vi "Chamber_control_Apr_ 2018.vi"() -> ()   [LabVIEW 2014]
doc: "This template is for the Queued Message Handler design pattern.\n\nThe Event Handling Loop generates messages based on user interface actions.\n\nThe Message Handling Loop processes messages generated by the Event Handling Loop, or by other messages. The messages are string values, so new messages can be added easily to the Message Cases case structure in the Message Handling Loop. Each message cluster can also provide an optional value for Message Data, which is a variant that can be converted to whatever message-specific data is required."
uses:
  <vilib>/Analysis/baseanly.llb/Mean (DBL).vi
  <vilib>/Instr/_visa.llb/VISA Configure Serial Port (Instr).vi
  Environmental Chamber LabVIEW and Instruments/Drivers and Software/Keithley 2100 Series/Public/Configure/Configure 2 Wire Resistance.vi
  <vilib>/Utility/file.llb/Read From Spreadsheet File (string).vi
  <vilib>/Utility/file.llb/Write To Spreadsheet File (string).vi
  Environmental Chamber LabVIEW and Instruments/Drivers and Software/LabVIEW 8.2 Drivers/keithley_24xx/Keithley 24XX/Public/Data/Read (Single Point).vi
  Environmental Chamber LabVIEW and Instruments/Drivers and Software/keithley_6430/Keithley 6430/Public/Data/Read (Single Point).vi
  Environmental Chamber LabVIEW and Instruments/Drivers and Software/keithley_6430/Keithley 6430/Keithley 6430.lvlib
  Environmental Chamber LabVIEW and Instruments/Drivers and Software/Keithley 2100 Series/Keithley 2100 Series.lvlib
  Environmental Chamber LabVIEW and Instruments/Drivers and Software/keithley_24xx/Keithley 24XX/Keithley 24XX.lvlib
  <vilib>/Analysis/NI_AALBase.lvlib
panel:
  out "Resistance":sgl format="%#_6e"
  in  "K2420 DC bias (V)":dbl=0.05
  in  "SYSTEM CONTROL":T1={"valve % open"=0.0, "Desired pressure"=0.0, "set Vapor sccm"=0.0, "set Gas sccm"=0.0, "Valve mode"=enum."% Open", "Pressure Mode"=enum."Abs. pressure", "analyte partial pressure"=23.8, "Actual"=0.0, "Read pressure (Torr)"=0.0, "Read vapor flow (sccm)"=0.0, "Read gas flow (sccm)"=0.0, "Save now"=FALSE, "Stop after seq."=TRUE, "Turbo pump\nauto on"=TRUE, "Integrate points"=0} caption="Pressure settings" {"Integrate points" min=0 max=100 step=1; "analyte partial pressure" min=0.0 max=100.0 step=5.0; "set Gas sccm" min=0 max=200 step=5; "set Vapor sccm" min=0 max=200 step=5; "Desired pressure" min=0.0 max=760.0 step=5.0; "valve % open" min=0.0 max=100.0 step=5.0 format="%#_2f"}
  in  "SAVE SAMPLE / ANALYTE NAMES":T2={"QCM1"="", "QCM2"="", "QCM3"="", "QCM4"="broken", "QCM5"="NOT WORKING", "QCM6"="", "SRS"="bareAu", "K-2420"="", "K-6430"="", "K-2100"="", "Gas"="NOT WORKING", "Vapor"="H2O", "Notes"=""} caption="Save samplffe names"
  in  "Clear all charts":bool
  out "K-6430":dbl(graph)
  out "K-2420":dbl(graph)
  out "File":path caption="DATA FILE"
  in  "Stop":bool
  out "QCM plot":T3(graph)
  out "K-2100":dbl(graph)
  out "State date/time":string caption="Program start time"
  out "J-KEM temp":dbl(graph)
  out "saving data?":bool
  out "pressure chart":dbl(graph)
  out "arduino qcm stack plot":T4(graph)
  in  "SEQUENCE":T5 {"preview" items=["pressure", "gas flow", "vapor flow", "bias"]}
  # "100"
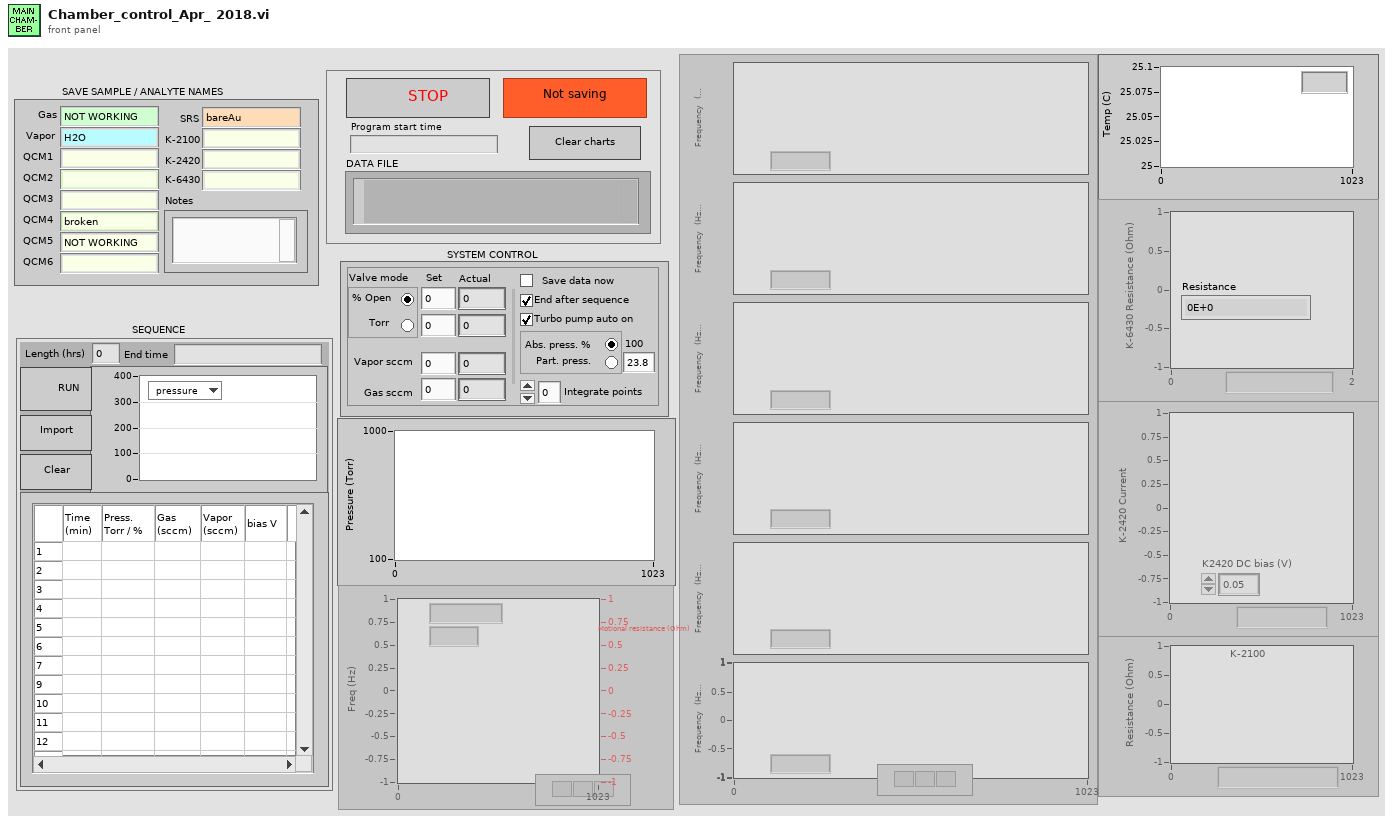
[diagram p1: front panel]
types:
  T1 = cluster{"valve % open":dbl, "Desired pressure":dbl, "set Vapor sccm":sgl, "set Gas sccm":sgl, "Valve mode":enum32{"% Open", "Torr "}, "Pressure Mode":enum32{"Abs. pressure", " Part. pressure"}, "analyte partial pressure":dbl, "Actual":dbl, "Read pressure (Torr)":dbl, "Read vapor flow (sccm)":dbl, "Read gas flow (sccm)":dbl, "Save now":bool, "Stop after seq.":bool, "Turbo pump\nauto on":bool, "Integrate points":i32}
  T2 = cluster{"QCM1":string, "QCM2":string, "QCM3":string, "QCM4":string, "QCM5":string, "QCM6":string, "SRS":string, "K-2420":string, "K-6430":string, "K-2100":string, "Gas":string, "Vapor":string, "Notes":string}
  T3 = cluster{"Frequency out":dbl, "Resistance out":dbl}
  T4 = cluster{"[0]":dbl, "[1]":dbl, "[2]":dbl, "[3]":dbl, "[4]":dbl, "[5]":dbl}
  T5 = cluster{"Run Sequence":bool, "User-defined\nsequence":string[][], "preview":u16, "Sequence\npreview":cluster{dbl[], dbl[]}[], "Clear sequence":bool, "Import sequence file":bool, "Length (hrs)":dbl, "End time":string}
  T6 = cluster{"Keithley 6430":bool, "J-KEM":bool, "Keithley 2420":bool, "Keithley 2100":bool, "SRS QCM":bool, "Pressure control":bool, "Arduino":bool}
  T7 = enum16{"open", "replace", "create", "open or create", "replace or create", "replace or create with confirmation"}
  T8 = cluster{"Arduino 1":refnum<visa-resource-name>, "Arduino 2":refnum<visa-resource-name>, "Arduino 3":refnum<visa-resource-name>, "Arduino 4":refnum<visa-resource-name>, "Arduino 5":refnum<visa-resource-name>, "Arduino 6":refnum<visa-resource-name>}
  T9 = enum8{"Enabled", "Disabled", "Disabled and Grayed Out"}
  T10 = cluster{"[0]":string, "[1]":string, "[2]":string, "[3]":string, "[4]":string, "[5]":string}
  T11 = cluster{"[0]":dbl, "[1]":dbl, "[2]":dbl, "[3]":dbl, "[4]":dbl, "[5]":dbl}[]
  T12 = cluster{"Frequency out":dbl, "Resistance out":dbl}[]
  T13 = cluster{"VISA resource name":refnum<visa-resource-name>, "error out":errorcluster, bool}
  T14 = cluster{"VISA resource name out":refnum<visa-resource-name>, "error out":errorcluster, bool}
  T15 = cluster{bool, "task out":refnum<k21>, "error out":errorcluster, "task out":refnum<k21>, "error out":errorcluster, "turbo pump":refnum<visa-resource-name>, "error out":errorcluster}
  T16 = cluster{bool, "task out":refnum<k21>, "error out":errorcluster, "task out":refnum<k21>, "error out":errorcluster, "VISA resource name out":refnum<visa-resource-name>, "error out":errorcluster}
  T17 = cluster{bool, "VISA resource name":refnum<visa-resource-name>, "error out":errorcluster}
  T18 = cluster{bool, "VISA resource name out":refnum<visa-resource-name>, "error out":errorcluster}
  T19 = cluster{bool, "VISA in":refnum<visa-resource-name>, "error out":errorcluster}
  T20 = cluster{bool, "VISA out":refnum<visa-resource-name>, "error out":errorcluster}
  T21 = cluster{"Arduino address":refnum<visa-resource-name>, "error in (no error)":errorcluster, "Arduino address 2":refnum<visa-resource-name>, "error in (no error) 2":errorcluster, "Arduino address 3":refnum<visa-resource-name>, "error in (no error) 3":errorcluster, "Arduino address 4":refnum<visa-resource-name>, "error in (no error) 4":errorcluster, "Arduino address 5":refnum<visa-resource-name>, "error in (no error) 5":errorcluster, "Arduino address 6":refnum<visa-resource-name>, "error in (no error) 6":errorcluster, "arduinos on?":bool}
  T22 = cluster{string[][], path, "data headers":string[]}
  T23 = cluster{"valve % open":dbl, "Desired pressure":dbl, "set Vapor sccm":sgl, "set Gas sccm":sgl, "Valve mode":enum32{"% Open", "Torr "}, "Pressure Mode":enum32{"Abs. pressure", " Part. pressure"}, "analyte partial pressure":dbl}
  T24 = cluster{"User-defined\nsequence":string[][], "Present (s)":dbl, "current  step # in":i32, "sequence end time in":timestamp}
  T25 = cluster{"current  step # in":i32, "sequence end time in":timestamp, "Boolean":bool}
  T26 = cluster{"press/RH/gas/vapor":cluster{"pressure":string, "RH":string, "gas flow":string, "vapor flow":string}, "Cluster":cluster{"Valve position (%)":dbl, "read pressure":dbl, "read vapor flow":dbl, "read gas flow":dbl}}
  T27 = cluster{"Boolean":bool, "task out":refnum<k21>, "error out":errorcluster, "task out":refnum<k21>, "error out":errorcluster, "VISA resource name out":refnum<visa-resource-name>, "error out":errorcluster}
  T28 = cluster{"t":string, "delta t":string, "p":string, "delta p":string}
  T29 = cluster{"pressure":string, "RH":string, "gas flow":string, "vapor flow":string}
  T30 = cluster{"Valve position (%)":dbl, "read pressure":dbl, "read vapor flow":dbl, "read gas flow":dbl}
  T31 = cluster{"Boolean":bool, "VISA resource name out":refnum<visa-resource-name>, "error out":errorcluster}
  T32 = cluster{"Boolean":bool, "VISA out":refnum<visa-resource-name>, "error out":errorcluster}
  T33 = cluster{"Boolean":bool, "Arduino address":refnum<visa-resource-name>, "error in (no error)":errorcluster, "Arduino address 2":refnum<visa-resource-name>, "error in (no error) 2":errorcluster, "Arduino address 3":refnum<visa-resource-name>, "error in (no error) 3":errorcluster, "Arduino address 4":refnum<visa-resource-name>, "error in (no error) 4":errorcluster, "Arduino address 5":refnum<visa-resource-name>, "error in (no error) 5":errorcluster, "Arduino address 6":refnum<visa-resource-name>, "error in (no error) 6":errorcluster}
  T34 = cluster{"arduino addresses out":cluster{"Boolean":bool, "Arduino address":refnum<visa-resource-name>, "error in (no error)":errorcluster, "Arduino address 2":refnum<visa-resource-name>, "error in (no error) 2":errorcluster, "Arduino address 3":refnum<visa-resource-name>, "error in (no error) 3":errorcluster, "Arduino address 4":refnum<visa-resource-name>, "error in (no error) 4":errorcluster, "Arduino address 5":refnum<visa-resource-name>, "error in (no error) 5":errorcluster, "Arduino address 6":refnum<visa-resource-name>, "error in (no error) 6":errorcluster}, cluster{bool, "VISA resource name out":refnum<visa-resource-name>, "error out":errorcluster}, "Address out":cluster{"Boolean":bool, "VISA resource name out":refnum<visa-resource-name>, "error out":errorcluster}, cluster{bool, "VISA resource name out":refnum<visa-resource-name>, "error out":errorcluster}, cluster{bool, "VISA resource name out":refnum<visa-resource-name>, "error out":errorcluster}, "SRS address out":cluster{"Boolean":bool, "VISA out":refnum<visa-resource-name>, "error out":errorcluster}}
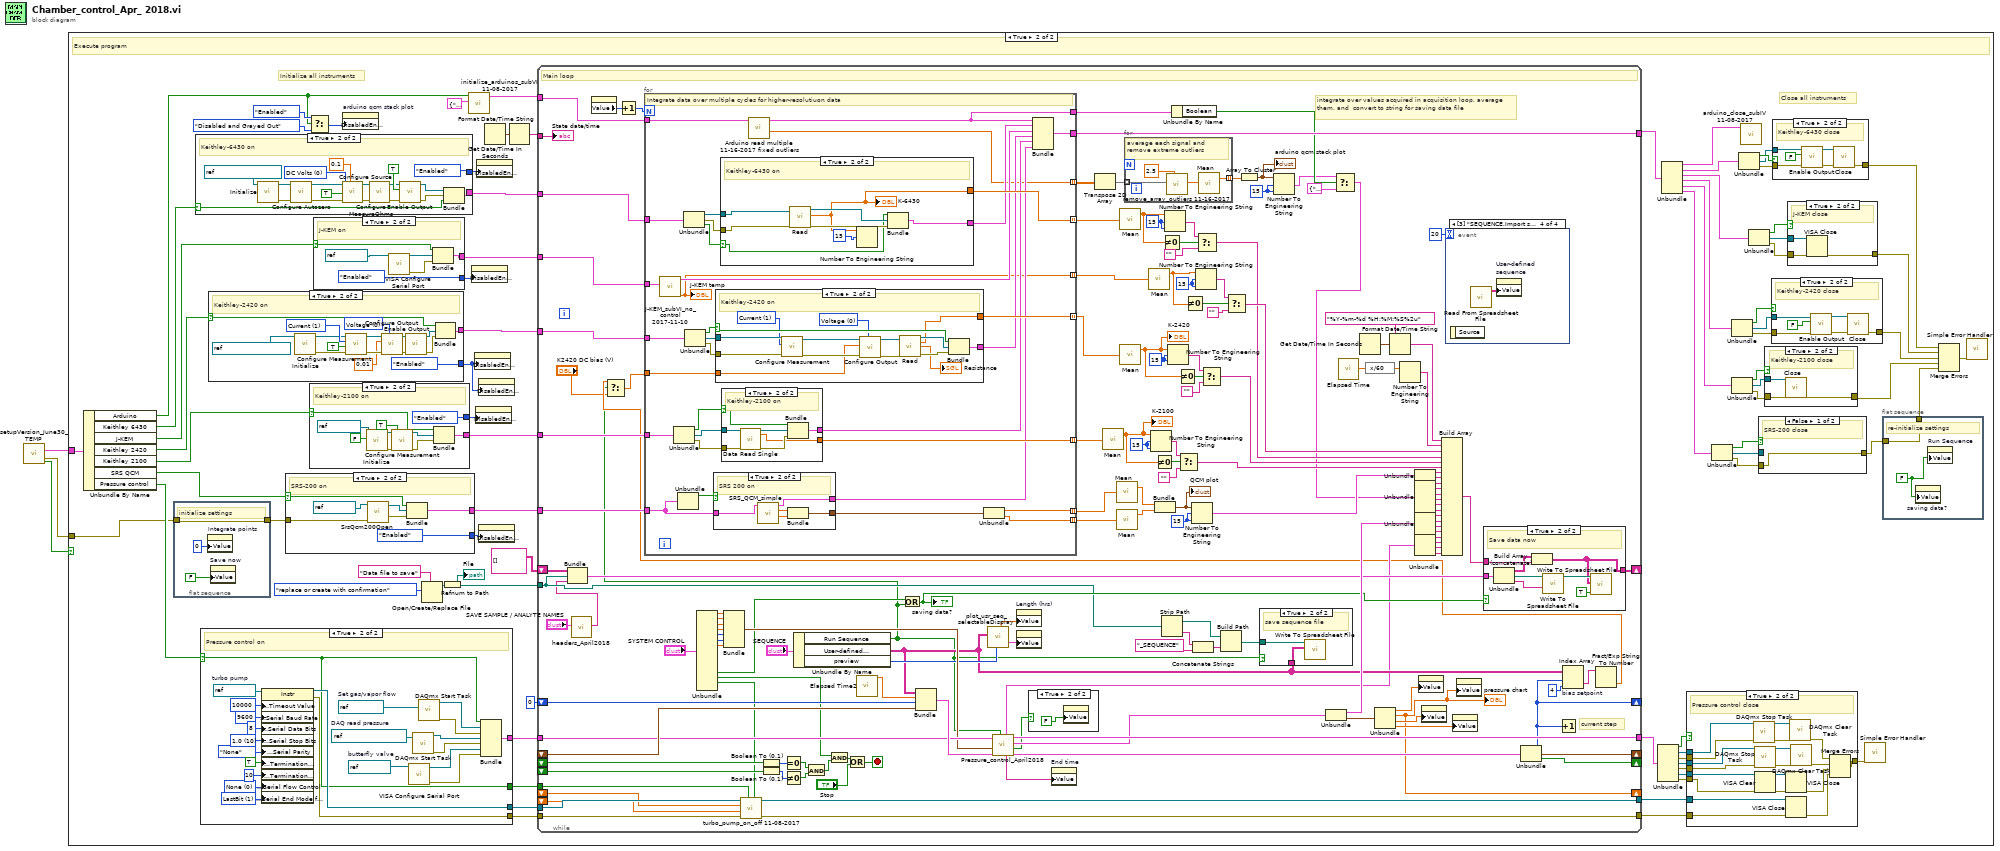
[diagram p0: block diagram]
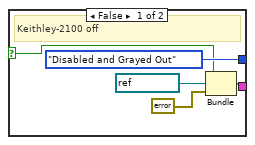
[diagram p4: hidden frame]
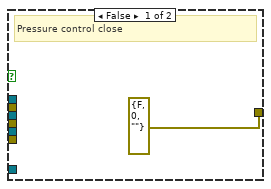
[diagram p5: hidden frame]
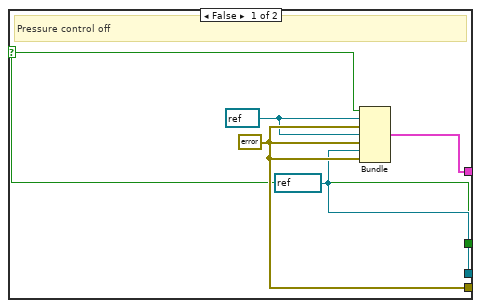
[diagram p6: hidden frame]
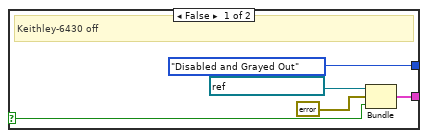
[diagram p8: hidden frame]
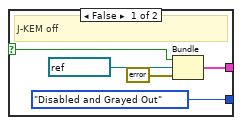
[diagram p10: hidden frame]
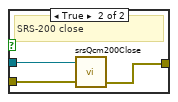
[diagram p11: hidden frame]
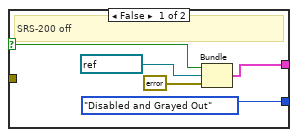
[diagram p12: hidden frame]
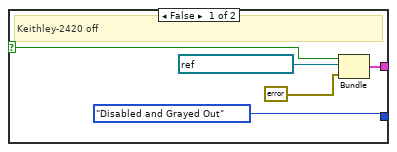
[diagram p14: hidden frame]
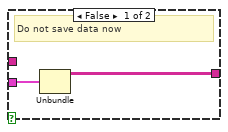
[diagram p16: hidden frame]
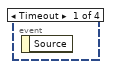
[diagram p17: hidden frame]
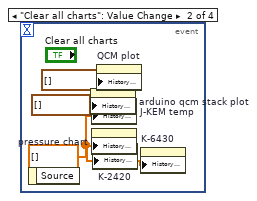
[diagram p18: hidden frame]
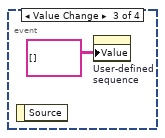
[diagram p19: hidden frame]
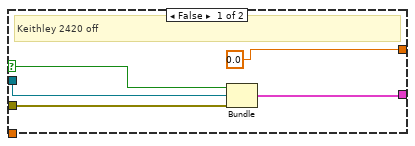
[diagram p20: hidden frame]
diagram:
  n1 = call "setupVersion_June30_TEMP.vi"() -> ("Instruments on/off"=w1:T6, "error IO"=w2:errorcluster, "OK"=w3:bool)  [unwired: 13 in]
  n2 = case shown="True" w3 {
    tunnel: w2 -> [_ w45]
    tunnel: w1 -> [_ w52]
    frame False {
      # "Cancel program"
    }
    frame True {
      # "Close all instruments"
      # "Initialize all instruments"
      # "Execute program"
      n3 = Unbundle By Name(w52) -> ("Arduino"=w24:bool, "Keithley 6430"=w51:bool, "J-KEM"=w50:bool, "Keithley 2420"=w49:bool, "Keithley 2100"=w48:bool, "SRS QCM"=w47:bool, "Pressure control"=w46:bool)
      n4 = flat-sequence {
        tunnel: [w83] -> w44
        tunnel: w45 -> [w83]
        frame #0 {
          # "initialize settings"
          n5 = property on="Integrate points" class="DigNum (strict)"("Value"=0) -> ()  [unwired: 2 in, 2 out]
          n6 = property on="Save now" class="Bool (strict)"("Value"=FALSE) -> ()  [unwired: 2 in, 2 out]
        }
      }
      n7 = case shown="True" w51 {
        selector: w51 -> [w161 w181]
        tunnel: [T9."Disabled and Grayed Out" ("Disabled") T9."Enabled" ("Disabled")] -> w30
        tunnel: [w160 w180] -> w28
        frame False {
          # "Keithley-6430 off"
          n8 = Bundle("VISA resource name"=refnum<visa-resource-name> "GPIB0::29::INSTR", "error out"=errorcluster {"status"=FALSE, "code"=0, "source"=""}, w161) -> (w160:T13)  [unwired: 1 in]
        }
        frame True {
          w168 = u16 0 items=["DC Volts", "DC Current"] ("Source Function (0: DC Volts)")
          # "Keithley-6430 on"
          n9 = call "Initialize.vi"("VISA resource name"=refnum<visa-resource-name> "GPIB2::19::INSTR") -> ("error out"=w174:errorcluster, "VISA resource name out"=w175:refnum<visa-resource-name>)  [unwired: 4 in, 5 out]
          n10 = call "Configure Autozero.vi"("error in (no error)"=w174, "VISA resource name"=w175) -> ("error out"=w171:errorcluster, "VISA resource name out"=w173:refnum<visa-resource-name>)  [unwired: 8 in]
          n11 = call "Configure Source.vi"("V-Source Level [V]"=0.1, "error in (no error)"=w171, "Auto Range (T:Enable)"=TRUE, "Source Function (0: DC Volts)"=w168, "VISA resource name"=w173) -> ("error out"=w170:errorcluster, "VISA resource name out"=w172:refnum<visa-resource-name>)  [unwired: 5 in]
          n12 = call "Configure MeasureOhms.vi"("error in (no error)"=w170, "VISA resource name"=w172) -> ("error out"=w179:errorcluster, "VISA resource name out"=w177:refnum<visa-resource-name>)  [unwired: 4 in, 4 out]
          n13 = call "Enable Output.vi"("error in (no error)"=w179, "Enable Output (F:Off)"=TRUE ("Output (F:Off)"), "VISA resource name"=w177) -> ("error out"=w166:errorcluster, "VISA resource name out"=w167:refnum<visa-resource-name>)  [unwired: 7 out]
          n14 = Bundle("VISA resource name out"=w167, "error out"=w166, w181) -> (w180:T14)  [unwired: 1 in]
        }
      }
      n15 = case shown="True" w46 {
        selector: w46 -> [w125 w131]
        tunnel: [w129 w132] -> w43
        tunnel: [w128 w130] -> w35
        tunnel: [w126 w133] -> w36
        tunnel: [w125 w131] -> w34
        frame False {
          w126 = refnum<visa-resource-name> refnum ("turbo pump")
          w127 = refnum<k21> refnum ("task out")
          w128 = errorcluster {"status"=FALSE, "code"=0, "source"=""} ("error out")
          # "Pressure control off"
          n16 = Bundle(w125, "task out"=w127, "error out"=w128, "task out"=w127, "error out"=w128, "turbo pump"=w126, "error out"=w128) -> (w129:T15)  [unwired: 1 in]
        }
        frame True {
          w137 = u16 1 items=["None", "LastBit", "TermChar"] ("Serial Settings:Serial End Mode for Reads")
          w135 = u16 0 items=["None", "XON/XOFF", "RTS/CTS", "XON/XOFF & RTS/CTS", "DTR/DSR", "XON/XOFF & DTR/DSR"] ("flow control (0:none)")
          w138 = u16 10 items=["1.0"=10, "1.5"=15, "2.0"=20] ("stop bits (10: 1 bit)")
          w134 = refnum<visa-resource-name> "COM7"  # turbo pump
          w150 = refnum<visa-resource-name> "COM5"  # butterfly valve
          w151 = refnum<k21> "Setflow"  # Set gas/vapor flow
          w152 = refnum<k21> "AllDaqReadings"  # DAQ read pressure
          # "Pressure control on"
          n17 = property class="Instr"(reference=w134, "General Settings:Timeout Value"=u32 10000 ("timeout (10sec)"), "Serial Settings:Serial Baud Rate"=u32 9600 ("baud rate (9600)"), "Serial Settings:Serial Data Bits"=u16 8 ("data bits (8)"), "Serial Settings:Serial Stop Bits"=w138, "Serial Settings:Serial Parity"=enum16{"None", "Odd", "Even", "Mark", "Space"}."None" ("parity (0:none)"), "Message Based Settings:Termination Character Enable"=TRUE ("Enable Termination\nChar (T)"), "Message Based Settings:Termination Character"=u8 10 ("termination char\n(0xA = '\\n' = LF)"), "Serial Settings:Serial Flow Control"=w135, "Serial Settings:Serial End Mode for Reads"=w137) -> (reference out=w133:refnum<visa-resource-name>, error out=w130:errorcluster)  [unwired: 1 in]
          n18 = call-poly "VISA Configure Serial Port"("VISA resource name"=w150) -> ("VISA resource name out"=w145:refnum<visa-resource-name>, "error out"=w144:errorcluster)  [unwired: 13 in]
          n19 = call <vilib>:"DAQmx Start Task.vi"("task/channels in"=w152) -> ("task out"=w147:refnum<k21>, "error out"=w146:errorcluster)  [unwired: 13 in]
          n20 = call <vilib>:"DAQmx Start Task.vi"("task/channels in"=w151) -> ("task out"=w149:refnum<k21>, "error out"=w148:errorcluster)  [unwired: 13 in]
          n21 = Bundle(w131, "task out"=w149, "error out"=w148, "task out"=w147, "error out"=w146, "VISA resource name out"=w145, "error out"=w144) -> (w132:T16)  [unwired: 1 in]
        }
      }
      n22 = case shown="True" w49 {
        selector: w49 -> [w224 w229]
        tunnel: [T9."Disabled and Grayed Out" ("Disabled") T9."Enabled" ("Disabled")] -> w9
        tunnel: [w222 w226] -> w27
        frame False {
          # "Keithley-2420 off"
          n23 = Bundle(w224, "VISA resource name"=refnum<visa-resource-name> "GPIB1::24::INSTR", "error out"=errorcluster {"status"=FALSE, "code"=0, "source"=""}) -> (w222:T17)  [unwired: 1 in]
        }
        frame True {
          w235 = u16 0 items=["Voltage", "Current"] ("Source Mode  (0: Voltage)")
          w240 = u16 1 items=["Volts", "Current", "Resistance"] ("Function (0: Volts)")
          # "Keithley-2420 on"
          n24 = call "Initialize.vi"("VISA resource name"=refnum<visa-resource-name> "GPIB1::24::INSTR") -> ("error out"=w230:errorcluster, "VISA resource name out"=w231:refnum<visa-resource-name>)  [unwired: 9 in]
          n25 = call "Configure Measurement.vi"("error in (no error)"=w230, "Enable Auto Range (T:Enable)"=TRUE, "Function (0: Volts)"=w240, "VISA resource name"=w231) -> ("error out"=w239:errorcluster, "VISA resource name out"=w238:refnum<visa-resource-name>)  [unwired: 6 in]
          n26 = call "Configure Output.vi"("Source Mode  (0: Voltage)"=w235, "error in (no error)"=w239, "Output Level (0)"=0.01 ("K2420 Applied Voltage (V) 2"), "VISA resource name"=w238) -> ("error out"=w237:errorcluster, "VISA resource name out"=w236:refnum<visa-resource-name>)  [unwired: 6 in]
          n27 = call "Enable Output.vi"("error in (no error)"=w237, "VISA resource name"=w236) -> ("error out"=w227:errorcluster, "VISA resource name out"=w228:refnum<visa-resource-name>)  [unwired: 8 in]
          n28 = Bundle(w229, "VISA resource name out"=w228, "error out"=w227) -> (w226:T18)  [unwired: 1 in]
        }
      }
      n29 = case shown="True" w47 {
        selector: w47 -> [w203 w209]
        tunnel: w44 -> [_ w212]
        tunnel: [T9."Disabled and Grayed Out" ("Disabled") T9."Enabled" ("Disabled")] -> w64
        tunnel: [w202 w208] -> w25
        frame False {
          # "SRS-200 off"
          n30 = Bundle(w203, "VISA in"=refnum<visa-resource-name> "COM6", "error out"=errorcluster {"status"=FALSE, "code"=0, "source"=""}) -> (w202:T19)  [unwired: 1 in]
        }
        frame True {
          # "SRS-200 on"
          n31 = call "SrsQcm200Open.vi"("error in"=w212, "VISA in"=refnum<visa-resource-name> "COM6") -> ("error out"=w207:errorcluster, "VISA out"=w210:refnum<visa-resource-name>)  [unwired: 3 in]
          n32 = Bundle(w209, "VISA out"=w210, "error out"=w207) -> (w208:T20)  [unwired: 1 in]
        }
      }
      n33 = Select(t=T9."Enabled" ("Disabled"), s=w24, f=T9."Disabled and Grayed Out" ("Disabled")) -> (s? t:f=w31:T9)
      n34 = case shown="True" w48 {
        selector: w48 -> [w93 w97]
        tunnel: [T9."Disabled and Grayed Out" ("Disabled") T9."Enabled" ("Disabled")] -> w61
        tunnel: [w90 w98] -> w26
        frame False {
          # "Keithley-2100 off"
          n35 = Bundle(w93, "VISA resource name out"=refnum<visa-resource-name> "K-2100", "error out"=errorcluster {"status"=FALSE, "code"=0, "source"=""}) -> (w90:T18)  [unwired: 1 in]
        }
        frame True {
          # "Keithley-2100 on"
          n36 = call "Initialize.vi"("VISA resource name"=refnum<visa-resource-name> "K-2100", "Reset? (T: Reset)"=FALSE) -> ("VISA resource name out"=w102:refnum<visa-resource-name>, "error out"=w101:errorcluster)  [unwired: 16 in]
          n37 = call-poly "Configure Measurement.vi"("VISA resource name"=w102, "error in (no error)"=w101, "Auto Range? (T: Auto)"=TRUE) -> ("VISA resource name out"=w96:refnum<visa-resource-name>, "error out"=w95:errorcluster)  [unwired: 15 in]
          n38 = Bundle(w97, "VISA resource name out"=w96, "error out"=w95) -> (w98:T18)  [unwired: 1 in]
        }
      }
      n39 = case shown="True" w50 {
        selector: w50 -> [w188 w194]
        tunnel: [w189 w195] -> w73
        tunnel: [T9."Disabled and Grayed Out" ("Disabled") T9."Enabled" ("Disabled")] -> w29
        frame False {
          # "J-KEM off"
          n40 = Bundle(w188, "VISA resource name"=refnum<visa-resource-name> "COM3", "error out"=errorcluster {"status"=FALSE, "code"=0, "source"=""}) -> (w189:T17)  [unwired: 1 in]
        }
        frame True {
          # "J-KEM on"
          n41 = call-poly "VISA Configure Serial Port"("VISA resource name"=refnum<visa-resource-name> "COM3") -> ("VISA resource name out"=w196:refnum<visa-resource-name>, "error out"=w193:errorcluster)  [unwired: 13 in]
          n42 = Bundle(w194, "VISA resource name out"=w196, "error out"=w193) -> (w195:T18)  [unwired: 1 in]
        }
      }
      n43 = property on="arduino qcm stack plot" class="WFChart (strict)"("DisabledEnum"=w31) -> ()  [unwired: 2 in, 2 out]
      n44 = Open/Create/Replace File(prompt="Data file to save", operation (0:open)=T7."replace or create with confirmation") -> (refnum out=w8:refnum<file>)  [unwired: 4 in, 2 out]
      n45 = Refnum to Path(1:w8) -> (0:w4:path)
      "File" <- w4
      n46 = call "initialize_arduinos_subVI 11-08-2017.vi"("arduino 1-6 addresses"=T8 {"Arduino 1"="COM25", "Arduino 2"="COM48", "Arduino 3"="COM21", "Arduino 4"="COM22", "Arduino 5"="COM23", "Arduino 6"="COM24"} ("Arduino COMs"), "arduinos on?"=w24) -> ("arduino addresses out"=w63:T21)  [unwired: 9 in]
      n47 = property on="J-KEM temp" class="WFChart (strict)"("DisabledEnum"=w29) -> ()  [unwired: 2 in, 2 out]
      n48 = property on="K-2420" class="WFChart (strict)"("DisabledEnum"=w9) -> ()  [unwired: 2 in, 2 out]
      n49 = property on="K-2100" class="WFChart (strict)"("DisabledEnum"=w61) -> ()  [unwired: 2 in, 2 out]
      n50 = property on="K-6430" class="WFChart (strict)"("DisabledEnum"=w30) -> ()  [unwired: 2 in, 2 out]
      n51 = property on="K2420 DC bias (V)" class="DigNum (strict)"("DisabledEnum"=w9) -> ()  [unwired: 2 in, 2 out]
      n52 = property on="QCM plot" class="WFChart (strict)"("DisabledEnum"=w64) -> ()  [unwired: 2 in, 2 out]
      n53 = Get Date/Time In Seconds() -> (seconds since 1Jan1904=w10:timestamp)
      n54 = Format Date/Time String(seconds (now)=w10) -> (date/time string=w60:string)  [unwired: 2 in]
      n55 = while {
        tunnel: w73 -> [w391]
        tunnel: w4 -> [w293]
        tunnel: w63 -> [w355]
        tunnel: w60 -> [w377]
        tunnel: w43 -> [w365]
        shift-right: [w351] -> _
        shift-left: 0 ("1st step") -> [w369]
        shift-right: [w374] -> _
        shift-left: _ -> [w372]
        shift-right: [w373] -> _
        shift-left: _ -> [w371]
        shift-left: _ -> [w370]
        tunnel: [w368] -> w56
        tunnel: w36 -> [w364]
        tunnel: w35 -> [w363]
        tunnel: w34 -> [w354]
        tunnel: [w361] -> w33
        tunnel: [w362] -> w32
        tunnel: w28 -> [w359]
        tunnel: w27 -> [w358]
        tunnel: w26 -> [w357]
        tunnel: w25 -> [w356]
        shift-right: [w305] -> _
        shift-left: _ -> [w353]
        shift-left: _ -> [w352]
        tunnel: [w254] -> w17
        shift-right: [w302] -> _
        shift-left: string[][] [] -> [w300]
        stop <- w383 stop-if-true
        w327 = i16 15 ("width (-)")
        w328 = i16 15 ("width (-)")
        w329 = i16 15 ("width (-)")
        w330 = i16 15 ("width (-)")
        w331 = i16 15 ("width (-)")
        w332 = i16 15 ("width (-)")
        # "current step"
        # "integrate over values acquired in acquisition loop, average them, and  convert to string for saving data file"
        # "Main loop"
        n56 = call "headers_April2018.vi"("Sample names"="SAVE SAMPLE / ANALYTE NAMES") -> ("data headers"=w247:string[])  [unwired: 10 in]
        n57 = Bundle(w300, w293, "data headers"=w247) -> (w297:T22)  [unwired: 1 in]
        n58 = property on="Integrate points" class="DigNum (strict)"() -> ("Value"=w299:i32)  [unwired: 2 in, 2 out]
        n59 = Increment(x=w299) -> (x+1=w334:i32)
        n60 = Unbundle("SYSTEM CONTROL") -> ("valve % open"=w320:dbl, "Desired pressure"=w319:dbl, "set Vapor sccm"=w318:sgl, "set Gas sccm"=w317:sgl, "Valve mode"=w316:enum32{"% Open", "Torr "}, "Pressure Mode"=w315:enum32{"Abs. pressure", " Part. pressure"}, "analyte partial pressure"=w314:dbl, "Save now"=w308:bool, "Stop after seq."=w307:bool, "Turbo pump\nauto on"=w306:bool)  [unwired: 5 out]
        n61 = Bundle("valve % open"=w320, "Desired pressure"=w319, "set Vapor sccm"=w318, "set Gas sccm"=w317, "Valve mode"=w316, "Pressure Mode"=w315, "analyte partial pressure"=w314) -> (w321:T23)  [unwired: 1 in]
        n62 = call "turbo_pump_on_off 11-08-2017.vi"("Turbo pump\nauto on"=w306, "pressure control on?"=w354, "error in (no error)"=w363, "read pressure"=w352, "read pressure 2"=w353, "VISA Refnum in"=w364) -> ("error out"=w362:errorcluster, "VISA Refnum out"=w361:refnum<visa-resource-name>)  [unwired: 4 in]
        n63 = Boolean To (0,1)(Boolean=w371) -> (0, 1=w387:i16)
        n64 = Boolean To (0,1)(Boolean=w370) -> (0, 1=w386:i16)
        n65 = Equal To 0?(x=w387) -> (x = 0?=w384:bool)
        n66 = Not Equal To 0?(x=w386) -> (x != 0?=w385:bool)
        n67 = Unbundle By Name("SEQUENCE") -> ("Run Sequence"=w242:bool, "User-defined\nsequence"=w294:string[][], "preview"=w312:u16)
        n68 = And(x=w384, y=w385) -> (x .and. y?=w382:bool)
        n69 = And(x=w307, y=w382) -> (x .and. y?=w381:bool)
        n70 = Or(x=w381, y="Stop") -> (x .or. y?=w383:bool)
        n71 = call "Elapsed Time2"() -> ("Present (s)"=w326:dbl)  [unwired: 12 in, 7 out]
        n72 = Or(x=w308, y=w242) -> (x .or. y?=w301:bool)
        "saving data?" <- w301
        n73 = Bundle("User-defined\nsequence"=w294, "Present (s)"=w326, "current  step # in"=w369, "sequence end time in"=w372) -> (w376:T24)  [unwired: 1 in]
        n74 = call "plot_usr_seq_selectableDisplay.vi"("Display"=w312, "User-defined sequence"=w294) -> ("Sequence Preview"=w311:cluster{dbl[], dbl[]}[], "seq length (hours)"=w298:dbl)  [unwired: 8 in]
        n75 = call "Pressure_control_April2018.vi"("Run Sequence"=w242, "user sequence, present (s) in, current step in, seq time in"=w376, "pressure parameters in"=w321, "pressure control on?/daq IDs/errors"=w365) -> ("current step # out, shift register time out, seq button on?"=w375:T25, "sequence over? USE THIS TO REINITIALIZE RUN SEQUENCE BUTTON SO PROGRAM ENDS"=w310:bool, "save press/RH/gasflow/vaporflow - read valve position/pressure/vaporflow/gasflow"=w367:T26, "pressure control on?/daq IDs/errors out"=w368:T27, "sequence end date/time string"=w304:string, "abs_t, delta_t, abs_p, delta_p"=w279:T28)  [unwired: 2 in]
        n76 = property on="Length (hrs)" class="DigNum (strict)"("Value"=w298) -> ()  [unwired: 2 in, 2 out]
        n77 = property on="Sequence\npreview" class="XYGraph (strict)"("Value"=w311) -> ()  [unwired: 2 in, 2 out]
        n78 = case shown="True" w310 {
          frame False {
          }
          frame True {
            n79 = property on="Run Sequence" class="Bool (strict)"("Value"=FALSE ("Run Sequence")) -> ()  [unwired: 2 in, 2 out]
          }
        }
        n80 = property on="End time" class="Str"("Value"=w304) -> ()  [unwired: 2 in, 2 out]
        n81 = Strip Path(path=w293) -> (stripped path=w296:path, name=w292:string)
        n82 = Concatenate Strings(w292, "_SEQUENCE" ("name or relative path")) -> (w290:string)
        n83 = Build Path(base path=w296, name or relative path=w290) -> (appended path=w295:path)
        n84 = case shown="True" w242 {
          tunnel: w295 -> [_ w394]
          tunnel: w294 -> [_ w393]
          frame False {
          }
          frame True {
            # "save sequence file"
            n85 = call-poly <vilib>:"Write To Spreadsheet File.vi"("2D data"=w393, "file path (dialog if empty)"=w394) -> ()  [unwired: 6 in, 1 out]
          }
        }
        n86 = Unbundle(w367) -> ("press/RH/gas/vapor"=w366:T29, "Cluster"=w325:T30)
        n87 = call "Elapsed Time"() -> ("Elapsed Time (s)"=w349:dbl)  [unwired: 12 in, 7 out]
        n88 = Get Date/Time In Seconds() -> (seconds since 1Jan1904=w392:timestamp)
        n89 = expression code="x/60"(w349) -> (w350:dbl)
        n90 = Unbundle(w325) -> ("Valve position (%)"=w324:dbl, "read pressure"=w305:dbl, "read vapor flow"=w323:dbl, "read gas flow"=w322:dbl)
        "pressure chart" <- w305
        n91 = Format Date/Time String(time format string (%c)="%Y-%m-%d %H:%M:%S%2u", seconds (now)=w392) -> (date/time string=w388:string)  [unwired: 1 in]
        n92 = Number To Engineering String ("elapsed time (min)")(4:w350) -> (0:w378:string)  [unwired: 3 in]
        n93 = Unbundle(w366) -> ("pressure"=w283:string, "RH"=w282:string, "gas flow"=w281:string, "vapor flow"=w280:string)
        n94 = Unbundle(w279) -> ("t"=w278:string, "delta t"=w277:string, "p"=w276:string, "delta p"=w275:string)
        n95 = property on="Actual" class="DigNum (strict)"("Value"=w324) -> ()  [unwired: 2 in, 2 out]
        n96 = property on="Read vapor flow (sccm)" class="DigNum (strict)"("Value"=w323) -> ()  [unwired: 2 in, 2 out]
        n97 = event shown="[3] \"SEQUENCE.Import sequence file\": Value Change" {
          selector: _ -> [_ _ _ _]
          dyn-events: _ -> [_ _ _ _]
          timeout: 20 -> [_ _ _ _]
          event Timeout {
            n98 = event-data() -> ()  [unwired: 1 in, 1 out]
          }
          event "Clear all charts": Value Change {
            w405 = dbl[] [] ("History Data")
            n99 = event-data() -> ()  [unwired: 1 in, 1 out]
            n100 = property on="arduino qcm stack plot" class="WFChart (strict)"("History Data"=T11 []) -> ()  [unwired: 2 in, 2 out]
            n101 = property on="J-KEM temp" class="WFChart (strict)"("History Data"=w405) -> ()  [unwired: 2 in, 2 out]
            n102 = property on="pressure chart" class="WFChart (strict)"("History Data"=w405) -> ()  [unwired: 2 in, 2 out]
            n103 = property on="K-2420" class="WFChart (strict)"("History Data"=w405) -> ()  [unwired: 2 in, 2 out]
            n104 = property on="QCM plot" class="WFChart (strict)"("History Data"=T12 []) -> ()  [unwired: 2 in, 2 out]
            n105 = property on="K-6430" class="WFChart (strict)"("History Data"=w405) -> ()  [unwired: 2 in, 2 out]
          }
          event "SEQUENCE.Clear sequence": Value Change {
            n106 = event-data() -> ()  [unwired: 1 in, 1 out]
            n107 = property on="User-defined\nsequence" class="Tbl (strict)"("Value"=string[][] []) -> ()  [unwired: 2 in, 2 out]
          }
          event "SEQUENCE.Import sequence file": Value Change {
            n108 = event-data() -> ()  [unwired: 1 in, 1 out]
            n109 = call-poly <vilib>:"Read From Spreadsheet File.vi"() -> ("all rows"=w409:string[][])  [unwired: 7 in, 4 out]
            n110 = property on="User-defined\nsequence" class="Tbl (strict)"("Value"=w409) -> ()  [unwired: 2 in, 2 out]
          }
        }
        n111 = property on="Read gas flow (sccm)" class="DigNum (strict)"("Value"=w322) -> ()  [unwired: 2 in, 2 out]
        n112 = property on="Read pressure (Torr)" class="DigNum (strict)"("Value"=w305) -> ()  [unwired: 2 in, 2 out]
        n113 = Unbundle(w375) -> ("current  step # in"=w351:i32, "sequence end time in"=w374:timestamp, "Boolean"=w373:bool)
        n114 = Increment(x=w351) -> ()  [unwired: 1 out]
        n115 = Index Array "bias setpoint"(array=w294, index (row)=w351, index (col)=4 ("disabled index (col)")) -> (element=w246:string)
        n116 = Fract/Exp String To Number(string=w246) -> (number=w245:dbl)  [unwired: 3 in, 1 out]
        n117 = Select(t=w245, s=w242, f="K2420 DC bias (V)") -> (s? t:f=w243:dbl)
        n118 = for {
          N: w334 -> [_]
          tunnel: w359 -> [w444]
          tunnel: w358 -> [w441]
          tunnel: w357 -> [w437]
          tunnel: w356 -> [w419]
          tunnel: w355 -> [w418]
          tunnel: w391 -> [w445]
          tunnel: [w432] -> w348 mode=indexing
          tunnel: [w431] -> w346 mode=indexing
          tunnel: [w417] -> w347 mode=indexing
          tunnel: [w430] -> w345 mode=indexing
          tunnel: [w428] -> w344 mode=indexing
          tunnel: [w427] -> w343 mode=indexing
          tunnel: [w416] -> w338 mode=indexing
          tunnel: [w421] -> w254
          tunnel: [w415] -> w252
          tunnel: w243 -> [w414]
          # "Integrate data over multiple cycles for higher-resolutiuon data"
          n119 = call "J-KEM_subVI_no_control 2017-11-10.vi"("Address in"=w445) -> ("Temp (C)"=w417:dbl, "Address out"=w425:T31)  [unwired: 9 in]
          "J-KEM temp" <- w417
          n120 = Unbundle(w437) -> (w436:bool, "VISA resource name out"=w435:refnum<visa-resource-name>, "error out"=w434:errorcluster)
          n121 = Unbundle(w419) -> (w420:bool)  [unwired: 2 out]
          n122 = Unbundle(w444) -> ("VISA resource name out"=w443:refnum<visa-resource-name>, "error out"=w433:errorcluster, w442:bool)
          n123 = Unbundle(w441) -> (w440:bool, "VISA resource name out"=w439:refnum<visa-resource-name>, "error out"=w438:errorcluster)
          n124 = case "SRS QCM" shown="True" w420 {
            tunnel: [w491 w497] -> w422
            tunnel: [T3 {"Frequency out"=0.0, "Resistance out"=0.0} ("freq, MR") w494] -> w429
            tunnel: w419 -> [w491 w493]
            frame False {
              # "SRS QCM off"
            }
            frame True {
              # "SRS 200 on"
              n125 = call "SRS_QCM_simple.vi"("SRS address in"=w493) -> ("Resistance out"=w496:dbl, "Frequency out"=w495:dbl, "SRS address out"=w497:T32)  [unwired: 8 in]
              n126 = Bundle("Frequency out"=w495, "Resistance out"=w496) -> (w494:T3)  [unwired: 1 in]
            }
          }
          n127 = case shown="True" w440 {
            selector: w440 -> [w450 w465]
            tunnel: [w447 w464] -> w424
            tunnel: w439 -> [w449 w458]
            tunnel: w438 -> [w448 w456]
            tunnel: [sgl 0.0 ("Resistance") w453] -> w431
            tunnel: w414 -> [_ w451]
            frame False {
              # "Keithley 2420 off"
              n128 = Bundle(w450, "VISA resource name out"=w449, "error out"=w448) -> (w447:T18)  [unwired: 1 in]
            }
            frame True {
              w454 = u16 1 items=["Volts", "Current", "Resistance"] ("Function (0: Volts)")
              w461 = u16 0 items=["Voltage", "Current"] ("Source Mode  (0: Voltage)")
              # "Keithley-2420 on"
              n129 = call "Configure Measurement.vi"("error in (no error)"=w456, "Function (0: Volts)"=w454, "VISA resource name"=w458) -> ("error out"=w455:errorcluster, "VISA resource name out"=w457:refnum<visa-resource-name>)  [unwired: 7 in]
              n130 = call "Configure Output.vi"("Source Mode  (0: Voltage)"=w461, "error in (no error)"=w455, "Output Level (0)"=w451, "VISA resource name"=w457) -> ("error out"=w459:errorcluster, "VISA resource name out"=w460:refnum<visa-resource-name>)  [unwired: 6 in]
              n131 = call-poly "Read.vi"("VISA resource name"=w460, "error in (no error)"=w459) -> ("VISA resource name out"=w463:refnum<visa-resource-name>, "Current"=w453:sgl, "Resistance"=→"Resistance":sgl, "error out"=w462:errorcluster)  [unwired: 7 in, 3 out]
              n132 = Bundle(w465, "VISA resource name out"=w463, "error out"=w462) -> (w464:T18)  [unwired: 1 in]
            }
          }
          n133 = case "Keithley 6430" shown="True" w442 {
            selector: w442 -> [w482 w485]
            tunnel: w443 -> [w481 w487]
            tunnel: [w480 w484] -> w426
            tunnel: w433 -> [w479 w486]
            tunnel: [0.0 ("K6340 Bias (V)") w483] -> w432
            frame False {
              # "Keithley-6430 off"
              n134 = Bundle(w482, "VISA resource name out"=w481, "error out"=w479) -> (w480:T18)  [unwired: 1 in]
            }
            frame True {
              # "Keithley-6430 on"
              n135 = call-poly "Read.vi"("error in (no error)"=w486, "VISA resource name"=w487) -> ("error out"=w488:errorcluster, "Measurement"=w483:dbl, "VISA resource name out"=w489:refnum<visa-resource-name>)  [unwired: 1 in, 6 out]
              "K-6430" <- w483
              n136 = Number To Engineering String(3:i16 15 ("width (-)"), 4:w483) -> ()  [unwired: 2 in, 1 out]
              n137 = Bundle(w485, "VISA resource name out"=w489, "error out"=w488) -> (w484:T18)  [unwired: 1 in]
            }
          }
          n138 = case shown="True" w436 {
            selector: w436 -> [w470 w475]
            tunnel: w435 -> [w468 w477]
            tunnel: w434 -> [w469 w476]
            tunnel: [w467 w472] -> w423
            tunnel: [0.0 ("Measurement") w471] -> w430
            frame False {
              # "Keithley-2100 off"
              n139 = Bundle(w470, "VISA resource name out"=w468, "error out"=w469) -> (w467:T18)  [unwired: 1 in]
            }
            frame True {
              # "Keithley-2100 on"
              n140 = call "Data Read Single.vi"("VISA resource name"=w477, "error in (no error)"=w476) -> ("VISA resource name out"=w474:refnum<visa-resource-name>, "Measurement"=w471:dbl, "error out"=w473:errorcluster)  [unwired: 15 in]
              n141 = Bundle(w475, "VISA resource name out"=w474, "error out"=w473) -> (w472:T18)  [unwired: 1 in]
            }
          }
          n142 = call "Arduino read multiple 11-16-2017 fixed outliers.vi"("arduino addresses in"=w418) -> ("freq out"=w416:dbl[], "arduino addresses out"=w415:T33)  [unwired: 8 in]
          n143 = Unbundle(w429) -> ("Frequency out"=w428:dbl, "Resistance out"=w427:dbl)
          n144 = Bundle("arduino addresses out"=w415, w426, "Address out"=w425, w424, w423, "SRS address out"=w422) -> (w421:T34)  [unwired: 1 in]
        }
        n145 = Transpose 2D Array(2D array=w338) -> (transposed array=w337:dbl[][])
        n146 = call-poly <vilib>:"Mean.vi"("X"=w345) -> ("mean"=w255:dbl)  [unwired: 1 out]
        "K-2100" <- w255
        n147 = call-poly <vilib>:"Mean.vi"("X"=w344) -> ("mean"=w342:dbl)  [unwired: 1 out]
        n148 = call-poly <vilib>:"Mean.vi"("X"=w343) -> ("mean"=w341:dbl)  [unwired: 1 out]
        n149 = call-poly <vilib>:"Mean.vi"("X"=w348) -> ("mean"=w262:dbl)  [unwired: 1 out]
        n150 = call-poly <vilib>:"Mean.vi"("X"=w346) -> ("mean"=w274:dbl)  [unwired: 1 out]
        "K-2420" <- w274
        n151 = for {
          tunnel: w337 -> [w412] mode=indexing
          tunnel: [w413] -> w336 mode=indexing
          # "average each signal and remove extreme outliers"
          n152 = call "remove_array_outliers 11-16-2017.vi"("n standard devs to filter"=2.5, "input array"=w412) -> ("filtered array out"=w411:dbl[])  [unwired: 9 in]
          n153 = call-poly <vilib>:"Mean.vi"("X"=w411) -> ("mean"=w413:dbl)  [unwired: 1 out]
        }
        n154 = call-poly <vilib>:"Mean.vi"("X"=w347) -> ("mean"=w267:dbl)  [unwired: 1 out]
        n155 = Number To Engineering String(2:w329, 3:w329, 4:w255) -> (0:w257:string)  [unwired: 1 in]
        n156 = Not Equal To 0?(x=w255) -> (x != 0?=w258:bool)
        n157 = Bundle("mean"=w342, "mean"=w341) -> (w340:cluster{"mean":dbl, "mean":dbl})  [unwired: 1 in]
        "QCM plot" <- w340
        n158 = Not Equal To 0?(x=w262) -> (x != 0?=w264:bool)
        n159 = Number To Engineering String(2:w332, 3:w332, 4:w262) -> (0:w261:string)  [unwired: 1 in]
        n160 = Number To Engineering String(2:w330, 3:w330, 4:w274) -> (0:w272:string)  [unwired: 1 in]
        n161 = Unbundle By Name(w252) -> ("Boolean"=w253:bool)
        n162 = Not Equal To 0?(x=w274) -> (x != 0?=w273:bool)
        n163 = Select(t=w257, s=w258, f="") -> (s? t:f=w256:string)
        n164 = Not Equal To 0?(x=w267) -> (x != 0?=w268:bool)
        n165 = Number To Engineering String(2:w327, 3:w327, 4:w340) -> (0:w339:cluster{"mean":string, "mean":string})  [unwired: 1 in]
        n166 = Number To Engineering String(2:w331, 3:w331, 4:w267) -> (0:w265:string)  [unwired: 1 in]
        n167 = Select(t=w261, s=w264, f="") -> (s? t:f=w260:string)
        n168 = Select(t=w272, s=w273, f="") -> (s? t:f=w271:string)
        n169 = Select(t=w265, s=w268, f="") -> (s? t:f=w266:string)
        n170 = Array To Cluster(array=w336) -> (cluster=w335:T4)
        "arduino qcm stack plot" <- w335
        n171 = Number To Engineering String(2:w328, 3:w328, 4:w335) -> (0:w251:T10)  [unwired: 1 in]
        n172 = Select(t=w251, s=w253, f=T10 {"[0]"="", "[1]"="", "[2]"="", "[3]"="", "[4]"="", "[5]"=""} ("Engineering string")) -> (s? t:f=w250:T10)
        n173 = Unbundle(w339) -> ("mean"=w379:string, "mean"=w389:string)
        n174 = Unbundle(w250) -> ("[0]"=w289:string, "[1]"=w288:string, "[2]"=w287:string, "[3]"=w286:string, "[4]"=w285:string, "[5]"=w284:string)
        n175 = Build Array(w388, w378, w266, w260, w271, w256, w379, w389, w289, w288, w287, w286, w285, w284, w283, w282, w281, w280, w278, w277, w276, w275) -> (w303:string[])
        n176 = case shown="True" w301 {
          tunnel: w303 -> [_ w404]
          tunnel: [w395 w401] -> w302
          tunnel: w297 -> [w396 w400]
          frame False {
            # "Do not save data now"
            n177 = Unbundle(w396) -> (w395:string[][])  [unwired: 2 out]
          }
          frame True {
            # "Save data now"
            n178 = Unbundle(w400) -> (w399:string[][], w398:path, "data headers"=w397:string[])
            n179 = Build Array (concatenate)(w399, w404) -> (w401:string[][])
            n180 = call-poly <vilib>:"Write To Spreadsheet File.vi"("1D data"=w397, "file path (dialog if empty)"=w398) -> ("new file path (Not A Path if cancelled)"=w402:path)  [unwired: 6 in]
            n181 = call-poly <vilib>:"Write To Spreadsheet File.vi"("append to file? (new file:F)"=TRUE, "2D data"=w401, "file path (dialog if empty)"=w402) -> ()  [unwired: 5 in, 1 out]
          }
        }
        "State date/time" <- w377
      }
      n182 = Unbundle(w56) -> ("Boolean"=w55:bool, "task out"=w42:refnum<k21>, "error out"=w41:errorcluster, "task out"=w40:refnum<k21>, "error out"=w39:errorcluster, "VISA resource name out"=w38:refnum<visa-resource-name>, "error out"=w37:errorcluster)
      n183 = Unbundle(w17) -> ("arduino addresses out"=w16:T33, w15:T18, "Address out"=w14:T31, w13:T18, w12:T18, "SRS address out"=w11:T32)
      n184 = case shown="True" w55 {
        tunnel: [errorcluster {"status"=FALSE, "code"=0, "source"=""} ("error out") w116] -> w59
        tunnel: w42 -> [_ w115]
        tunnel: w41 -> [_ w114]
        tunnel: w40 -> [_ w113]
        tunnel: w39 -> [_ w110]
        tunnel: w38 -> [_ w111]
        tunnel: w37 -> [_ w112]
        tunnel: w33 -> [_ w107]
        tunnel: w32 -> [_ w106]
        frame False {
          # "Pressure control close"
        }
        frame True {
          # "Pressure control close"
          n185 = call <vilib>:"DAQmx Stop Task.vi"("task/channels in"=w115, "error in"=w114) -> ("task out"=w122:refnum<k21>, "error out"=w121:errorcluster)  [unwired: 12 in]
          n186 = call <vilib>:"DAQmx Stop Task.vi"("task/channels in"=w113, "error in"=w110) -> ("task out"=w123:refnum<k21>, "error out"=w124:errorcluster)  [unwired: 12 in]
          n187 = VISA Clear(VISA resource name=w111, error in (no error)=w112) -> (VISA resource name out=w120:refnum<visa-resource-name>, error out=w119:errorcluster)
          n188 = VISA Close(VISA resource name=w107, error in (no error)=w106) -> (error out=w108:errorcluster)
          n189 = VISA Close(VISA resource name=w120, error in (no error)=w119) -> (error out=w109:errorcluster)
          n190 = call <vilib>:"DAQmx Clear Task.vi"("task in"=w122, "error in"=w121) -> ("error out"=w118:errorcluster)  [unwired: 13 in]
          n191 = call <vilib>:"DAQmx Clear Task.vi"("task in"=w123, "error in"=w124) -> ("error out"=w117:errorcluster)  [unwired: 13 in]
          n192 = Merge Errors(w118, w117, w109, w108) -> (w116:errorcluster)
        }
      }
      n193 = Unbundle(w11) -> ("Boolean"=w75:bool, "VISA out"=w74:refnum<visa-resource-name>, "error out"=w20:errorcluster)
      n194 = Unbundle(w13) -> (w78:bool, "VISA resource name out"=w77:refnum<visa-resource-name>, "error out"=w76:errorcluster)
      n195 = Unbundle(w12) -> (w23:bool, "VISA resource name out"=w22:refnum<visa-resource-name>, "error out"=w21:errorcluster)
      n196 = Unbundle(w15) -> (w68:bool, "VISA resource name out"=w67:refnum<visa-resource-name>, "error out"=w66:errorcluster)
      n197 = call "arduino_close_subIV 11-08-2017.vi"("arduino addresses out"=w16) -> ()  [unwired: 11 in]
      n198 = Unbundle(w14) -> ("Boolean"=w72:bool, "VISA resource name out"=w71:refnum<visa-resource-name>, "error out"=w70:errorcluster)
      n199 = case shown="False" w75 {
        tunnel: [w198 w201] -> w19
        tunnel: w74 -> [_ w200]
        tunnel: w20 -> [w198 w199]
        frame False {
          # "SRS-200 close"
        }
        frame True {
          # "SRS-200 close"
          n200 = call "srsQcm200Close.vi"("error in"=w199, "Visa in"=w200) -> ("error out"=w201:errorcluster)  [unwired: 3 in]
        }
      }
      n201 = case shown="True" w23 {
        tunnel: w22 -> [_ w89]
        tunnel: w21 -> [w86 w88]
        tunnel: [w86 w87] -> w62
        frame False {
          # "Keithley-2100 close"
        }
        frame True {
          # "Keithley-2100 close"
          n202 = call "Close.vi"("VISA resource name"=w89, "error in (no error)"=w88) -> ("error out"=w87:errorcluster)  [unwired: 17 in]
        }
      }
      n203 = case shown="True" w78 {
        tunnel: w77 -> [_ w217]
        tunnel: w76 -> [w214 w216]
        tunnel: [w214 w215] -> w79
        frame False {
          # "Keithley-2420 close"
        }
        frame True {
          # "Keithley-2420 close"
          n204 = call "Enable Output.vi"("error in (no error)"=w216, "Enable Output (T: Enable)"=FALSE, "VISA resource name"=w217) -> ("error out"=w218:errorcluster, "VISA resource name out"=w220:refnum<visa-resource-name>)  [unwired: 7 in]
          n205 = call "Close.vi"("error in (no error)"=w218, "VISA resource name"=w220) -> ("error out"=w215:errorcluster)  [unwired: 9 in]
        }
      }
      n206 = case shown="True" w68 {
        tunnel: w67 -> [_ w155]
        tunnel: w66 -> [w153 w154]
        tunnel: [w153 w156] -> w65
        frame False {
          # "Keithley-6430 close"
        }
        frame True {
          # "Keithley-6430 close"
          n207 = call "Enable Output.vi"("error in (no error)"=w154, "Enable Output (F:Off)"=FALSE ("Output (F:Off)"), "VISA resource name"=w155) -> ("error out"=w157:errorcluster, "VISA resource name out"=w158:refnum<visa-resource-name>)  [unwired: 7 out]
          n208 = call "Close.vi"("error in (no error)"=w157, "VISA resource name"=w158) -> ("error out"=w156:errorcluster)  [unwired: 9 out]
        }
      }
      n209 = case shown="True" w72 {
        tunnel: w71 -> [_ w186]
        tunnel: w70 -> [w183 w185]
        tunnel: [w183 w184] -> w69
        frame False {
          # "J-KEM close"
        }
        frame True {
          # "J-KEM close"
          n210 = VISA Close(VISA resource name=w186, error in (no error)=w185) -> (error out=w184:errorcluster)
        }
      }
      n211 = call <vilib>:"Simple Error Handler.vi"("error in (no error)"=w59) -> ()  [unwired: 4 in, 5 out]
      n212 = flat-sequence {
        tunnel: w19 -> [w85]
        tunnel: [w85] -> w18
        frame #0 {
          w84 = FALSE ("saving data?")
          # "re-initialize settings"
          n213 = property on="saving data?" class="Bool (strict)"("Value"=w84) -> ()  [unwired: 2 in, 2 out]
          n214 = property on="Run Sequence" class="Bool (strict)"("Value"=w84) -> ()  [unwired: 2 in, 2 out]
        }
      }
      n215 = Merge Errors(w65, w69, w79, w62, w18) -> (w80:errorcluster)
      n216 = call <vilib>:"Simple Error Handler.vi"("error in (no error)"=w80) -> ()  [unwired: 4 in, 5 out]
    }
  }
